vi "Qmax.vi"(11 "Qmax":dbl) -> (3 "18 punti out":T1)   [LabVIEW 2019]
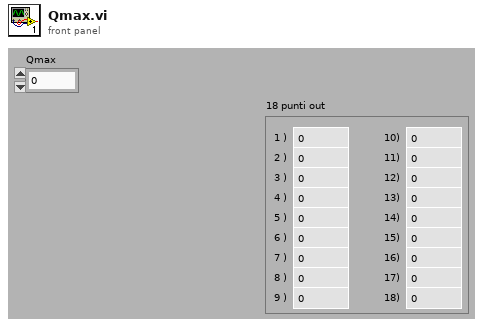
[diagram p1: front panel]
types:
  T1 = cluster{"1 )":dbl, "2 )":dbl, "3 )":dbl, "4 )":dbl, "5 )":dbl, "6 )":dbl, "7 )":dbl, "8 )":dbl, "9 )":dbl, "10)":dbl, "11)":dbl, "12)":dbl, "13)":dbl, "14)":dbl, "15)":dbl, "16)":dbl, "17)":dbl, "18)":dbl}
  T2 = cluster{"[0]":dbl, "[1]":dbl, "[2]":dbl, "[3]":dbl, "[4]":dbl, "[5]":dbl, "[6]":dbl, "[7]":dbl, "[8]":dbl, "[9]":dbl, "[10]":dbl, "[11]":dbl, "[12]":dbl, "[13]":dbl, "[14]":dbl, "[15]":dbl, "[16]":dbl, "[17]":dbl}
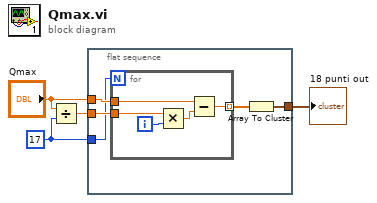
[diagram p0: block diagram]
diagram:
  w1 = 17
  n1 = Divide(x="Qmax", y=w1) -> (x/y=w4:dbl)
  n2 = flat-sequence {
    tunnel: w4 -> [w9]
    tunnel: [w7] -> w3
    tunnel: "Qmax" -> [w6]
    tunnel: w1 -> [w5]
    frame #0 {
      n3 = for {
        N: w5 -> [_]
        tunnel: w9 -> [w14]
        tunnel: [w11] -> w8 mode=indexing
        tunnel: w6 -> [w10]
        i -> [w13]
        n4 = Multiply(x=w14, y=w13) -> (x*y=w12:dbl)
        n5 = Subtract(x=w10, y=w12) -> (x-y=w11:dbl)
      }
      n6 = Array To Cluster(array=w8) -> (cluster=w7:T2)
    }
  }
  "18 punti out" <- w3
